vi "QueVariant.vi"(6 "MODE(GET)":T1=enum."Get", 7 "最大キューサイズ（-1, 無制限）":i32=-1, 8 "error in":errorcluster, 10 "Que名称":string, 11 "queVariant(in)":refnum<queue>) -> (0 "error out":errorcluster, 3 "queVariant":refnum<queue>)   [LabVIEW 2016]
uses:
  QueueMakeMode.ctl
  Event/Ctl/EventVariantData.ctl
panel:
  out "取得済みQueue":string[](array[string])
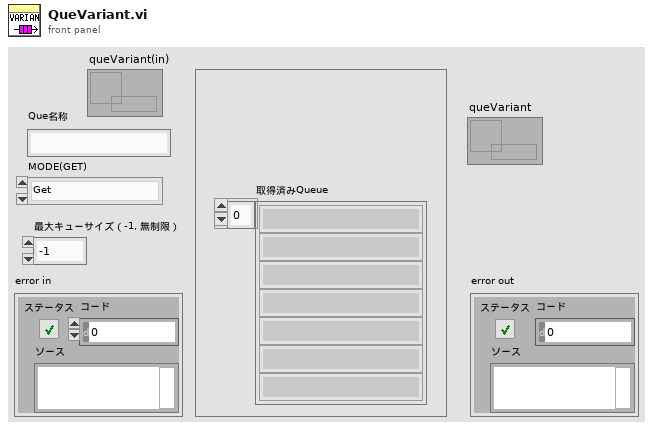
[diagram p1: front panel]
types:
  T1 = typedef "QueueMakeMode.ctl" = enum16{"Create", "Get", "Release", "ReleaseAll"}
  T2 = typedef "EventVariantData.ctl" = cluster{"コマンド":string, "バリアント":variant}
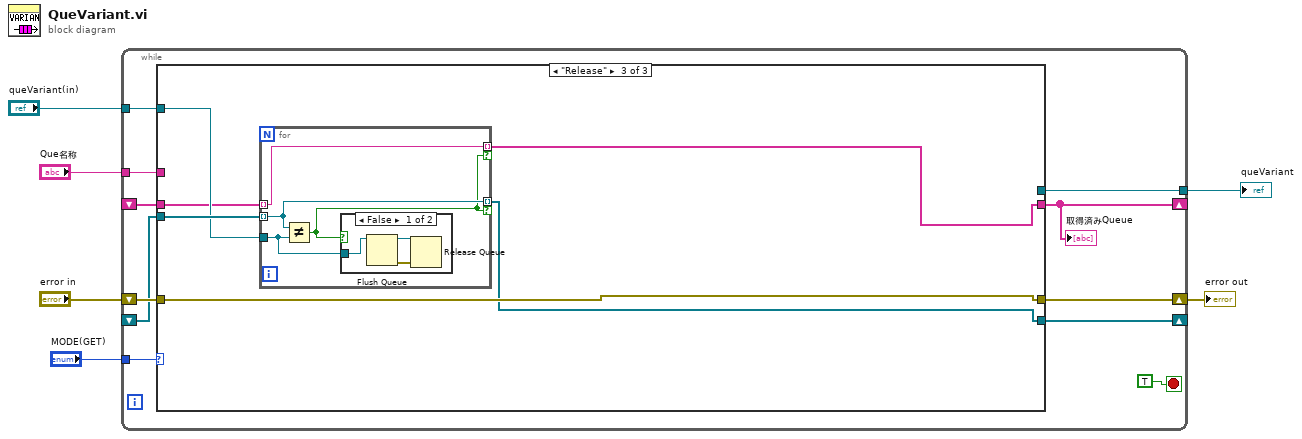
[diagram p0: block diagram]
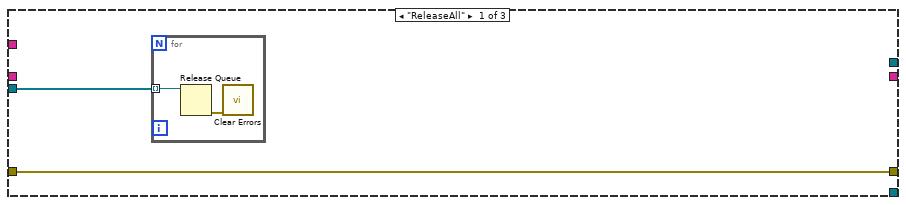
[diagram p2: hidden frame]
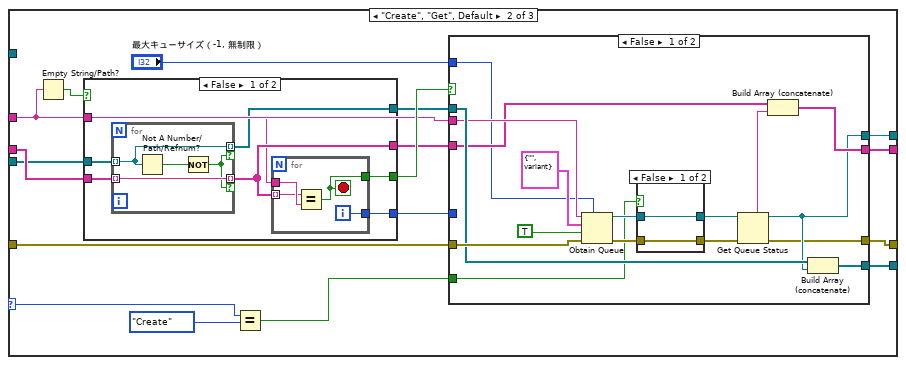
[diagram p3: hidden frame]
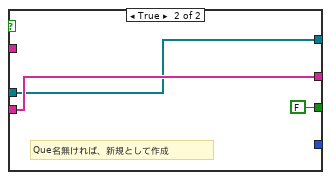
[diagram p4: hidden frame]
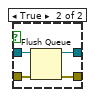
[diagram p5: hidden frame]
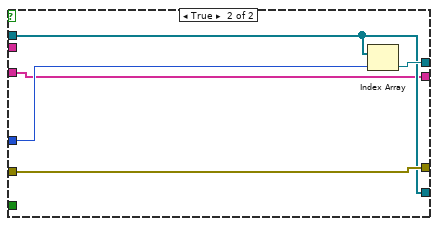
[diagram p6: hidden frame]
diagram:
  n1 = while {
    tunnel: "MODE(GET)" -> [w16]
    shift-right: [w15] -> w3
    shift-left: "error in" -> [w14]
    shift-right: [w13] -> _
    shift-left: _ -> [w11]
    tunnel: "Que名称" -> [w10]
    tunnel: [w9] -> w2
    shift-right: [w8] -> _
    shift-left: _ -> [w12]
    tunnel: "queVariant(in)" -> [w7]
    stop <- TRUE stop-if-true
    n2 = case shown="\"Release\"" w16 {
      selector: w16 -> [_ w27 _]
      tunnel: [w18 w38 w87] -> w15
      tunnel: w14 -> [w18 w37 w87]
      tunnel: [_ w33 w86] -> w13
      tunnel: w12 -> [_ w30 w88]
      tunnel: w11 -> [w19 w29 w90]
      tunnel: w10 -> [_ w23 _]
      tunnel: [_ w35 _] -> w9
      tunnel: [_ w32 w85] -> w8
      tunnel: w7 -> [_ _ w89]
      frame "ReleaseAll" {
        n3 = for {
          tunnel: w19 -> [w21] mode=indexing
          n4 = Release Queue(queue=w21) -> (error out=w20:errorcluster)  [unwired: 2 in, 2 out]
          n5 = call <vilib>:"Clear Errors.vi"("error in (no error)"=w20) -> ()  [unwired: 5 in, 2 out]
        }
      }
      frame "Create", "Get", Default {
        n6 = Empty String/Path?(string/path=w23) -> (empty?=w22:bool)
        n7 = case shown="FALSE" w22 {
          tunnel: [w45 FALSE] -> w36
          tunnel: [w44 _] -> w34
          tunnel: [w43 w56] -> w31
          tunnel: w30 -> [w42 w56]
          tunnel: w29 -> [w41 w55]
          tunnel: [w40 w55] -> w28
          tunnel: w23 -> [w39 _]
          frame False {
            n8 = for {
              tunnel: [w49] -> w43 mode=indexing if=w46
              tunnel: w42 -> [w49] mode=indexing
              tunnel: [w48] -> w40 mode=indexing if=w46
              tunnel: w41 -> [w48] mode=indexing
              n9 = Not A Number/Path/Refnum?(number/path/refnum=w48) -> (NaN/Path/Refnum?=w47:bool)
              n10 = Not(x=w47) -> (.not. x?=w46:bool)
            }
            n11 = for {
              tunnel: w39 -> [w53]
              tunnel: w43 -> [w50] mode=indexing
              tunnel: [w52] -> w44
              tunnel: [w51] -> w45
              i -> [w52]
              stop <- w51 stop-if-true
              n12 = Equal?(x=w50, y=w53) -> (x = y?=w51:bool)
            }
          }
          frame True {
            # "Que名無ければ、新規として作成"
          }
        }
        n13 = Equal?(x=w27, y=QueueMakeMode."Create" ("MODE(GET)")) -> (x = y?=w26:bool)
        n14 = case shown="FALSE" w36 {
          tunnel: [w58 w84] -> w38
          tunnel: w37 -> [w73 w84]
          tunnel: [w60 w82] -> w35
          tunnel: w23 -> [w68 _]
          tunnel: w28 -> [w70 w81]
          tunnel: w34 -> [_ w83]
          tunnel: [w69 w81] -> w33
          tunnel: w31 -> [w67 w80]
          tunnel: [w66 w80] -> w32
          tunnel: "最大キューサイズ（-1, 無制限）" -> [w64 _]
          tunnel: w26 -> [w62 _]
          frame False {
            n15 = Obtain Queue(max queue size (-1, unlimited)=w64, name (unnamed)=w68, element data type=T2 {"コマンド"="", "バリアント"=variant}, create if not found? (T)=TRUE, error in (no error)=w73) -> (queue out=w71:refnum<queue>, error out=w72:errorcluster)  [unwired: 1 out]
            n16 = case shown="FALSE" w62 {
              tunnel: [w74 w79] -> w59
              tunnel: w72 -> [w74 w78]
              tunnel: w71 -> [w75 w77]
              tunnel: [w75 w76] -> w61
              frame False {
              }
              frame True {
                n17 = Flush Queue(queue=w77, error in (no error)=w78) -> (queue out=w76:refnum<queue>, error out=w79:errorcluster)  [unwired: 1 out]
              }
            }
            n18 = Get Queue Status(queue=w61, error in (no error)=w59) -> (queue out=w60:refnum<queue>, queue name=w57:string, error out=w58:errorcluster)  [unwired: 1 in, 5 out]
            n19 = Build Array (concatenate)(w67, w57) -> (w66:string[])
            n20 = Build Array (concatenate)(w70, w60) -> (w69:refnum<queue>[])
          }
          frame True {
            n21 = Index Array(array=w81, index=w83) -> (element=w82:refnum<queue>)
          }
        }
      }
      frame "Release" {
        n22 = for {
          tunnel: [w94] -> w86 mode=indexing if=w91
          tunnel: w90 -> [w94] mode=indexing
          tunnel: w89 -> [w93]
          tunnel: [w92] -> w85 mode=indexing if=w91
          tunnel: w88 -> [w92] mode=indexing
          n23 = Not Equal?(x=w94, y=w93) -> (x != y?=w91:bool)
          n24 = case shown="FALSE" w91 {
            tunnel: w93 -> [w97 _]
            frame False {
              n25 = Flush Queue(queue=w97) -> (queue out=w96:refnum<queue>, error out=w95:errorcluster)  [unwired: 1 in, 1 out]
              n26 = Release Queue(queue=w96, error in (no error)=w95) -> ()  [unwired: 1 in, 3 out]
            }
            frame True {
            }
          }
        }
      }
    }
    "取得済みQueue" <- w8
  }
  "error out" <- w3
  "queVariant" <- w2
